vi "KI_schedule.vi"(4 "KI_max":fxp<+/-,64,32> format="%#_42g", 6 "KI_min":fxp<+/-,64,32>, 8 "enable":bool, 9 "KI_slope":fxp<+/-,32,16>, 10 "KI_o":fxp<+/-,32,16>, 11 "dfl_error":fxp<+/-,32,16> format="%#_21g") -> (2 "KI_sched":fxp<+/-,64,32>)   [LabVIEW 2017]
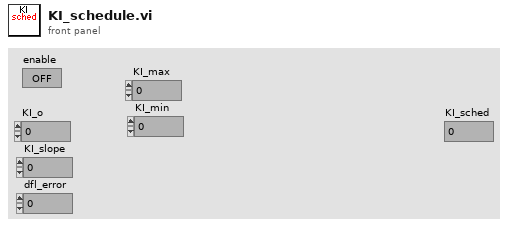
[diagram p1: front panel]
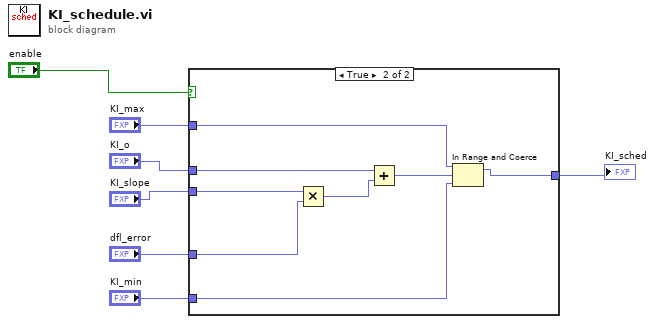
[diagram p0: block diagram]
diagram:
  n1 = case shown="True" "enable" {
    tunnel: "KI_o" -> [w8 w15]
    tunnel: "KI_slope" -> [_ w14]
    tunnel: "dfl_error" -> [_ w13]
    tunnel: [w8 w11] -> w3
    tunnel: "KI_max" -> [_ w10]
    tunnel: "KI_min" -> [_ w9]
    frame False {
    }
    frame True {
      n2 = Multiply(x=w14, y=w13) -> (x*y=w16:fxp<+/-,64,32>)
      n3 = Add(x=w15, y=w16) -> (x+y=w12:fxp<+/-,64,32>)
      n4 = In Range and Coerce(upper limit=w10, x=w12, lower limit=w9) -> (coerced(x)=w11:fxp<+/-,64,32>)  [unwired: 1 out]
    }
  }
  "KI_sched" <- w3
